vi "getmaxPDF.vi"(6 "addr/port":cluster{"address":string, "port":i32}={"address"="127.0.0.1", "port"=31415}, 8 "error in (no error)":errorcluster) -> (0 "error out":errorcluster, 3 "maxparams":cluster{"x0":dbl, "A":dbl, "B":dbl})   [LabVIEW 2015]
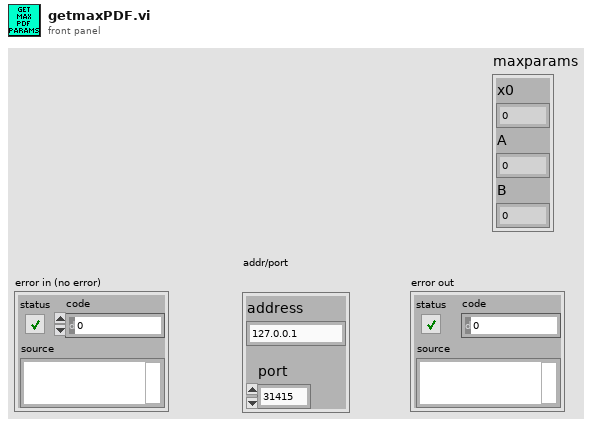
[diagram p1: front panel]
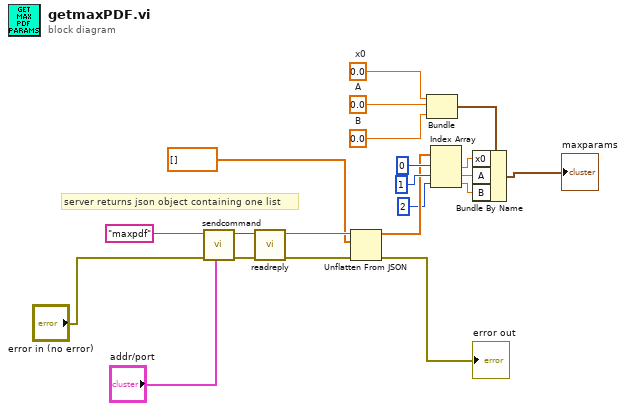
[diagram p0: block diagram]
diagram:
  w4 = 0.0  # B
  w8 = 0.0  # A
  w9 = 0.0  # x0
  # "server returns json object containing one list"
  n1 = call "sendcommand.vi"("addr/port"="addr/port", "error in (no error)"="error in (no error)", "command"="maxpdf") -> ("error out"=w17:errorcluster, "connection ID out"=w18:refnum<k5>)  [unwired: 6 in, 1 out]
  n2 = call "readreply.vi"("error in (no error)"=w17, "connection ID"=w18) -> ("error out"=w16:errorcluster, "data out"=w14:string)  [unwired: 8 in]
  n3 = Unflatten From JSON(JSON string=w14, type and defaults=dbl[] [] ("Array"), error in (no error)=w16) -> (value=w10:dbl[], error out=→"error out":errorcluster)  [unwired: 4 in]
  n4 = Bundle("x0"=w9, "A"=w8, "B"=w4) -> (w7:cluster{"x0":dbl, "A":dbl, "B":dbl})  [unwired: 1 in]
  n5 = Index Array(array=w10, index #1=0 ("index"), index #2=1 ("index"), index #3=2 ("index")) -> (element #1=w6:dbl, element #2=w5:dbl, element #3=w3:dbl)
  n6 = Bundle By Name(cluster=w7, "x0"=w6, "A"=w5, "B"=w3) -> (→"maxparams":cluster{"x0":dbl, "A":dbl, "B":dbl})
